vi "RecordWave_and_WAVFile.vi"() -> ()   [LabVIEW 2016]
uses:
  WaveIO.llb/SoundHandle.ctl
panel:
  in  "Write CSV":bool
  out "bufferTime [µs]":dbl format="%#_6f"
  out "Time[sec]":dbl
  out "About":string
  in  "Stop File":bool
  in  "time to record":u32=1000 min=10 max=60000 step=10
  out "bufNo":i32=337
  out "Sound Handle IN":T1={"DeviceID"=0, "Samples/buf"=2205, "Sampl rate"=44100, "Bits/sample"=16, "Channels"=2, "Opened"=TRUE}
  in  "Record File":bool
  in  "Name of WAV File":path=path "soundcard_data.wav"
  in  "card #":u32
  out "Device Names":string[](array[string])
  out "Number of Input Devices":i32=3
  out "error out":errorcluster
  out "Rec Error":errorcluster
  in  "Format":cluster{"Rate":i32, "Bits":i32, "Channels":i32}={"Rate"=44100, "Bits"=16, "Channels"=2}
  in  "Buffer":T2={"# buffers"=10, "Buffer size"=50, "unit (ms)"=enum."time (ms)"}
  out "Waveform Graph":i32[][](graph)
  in  "Stop":bool=TRUE
  # "msec"
  # "ONLY for Information\nHas no effect in the code !"
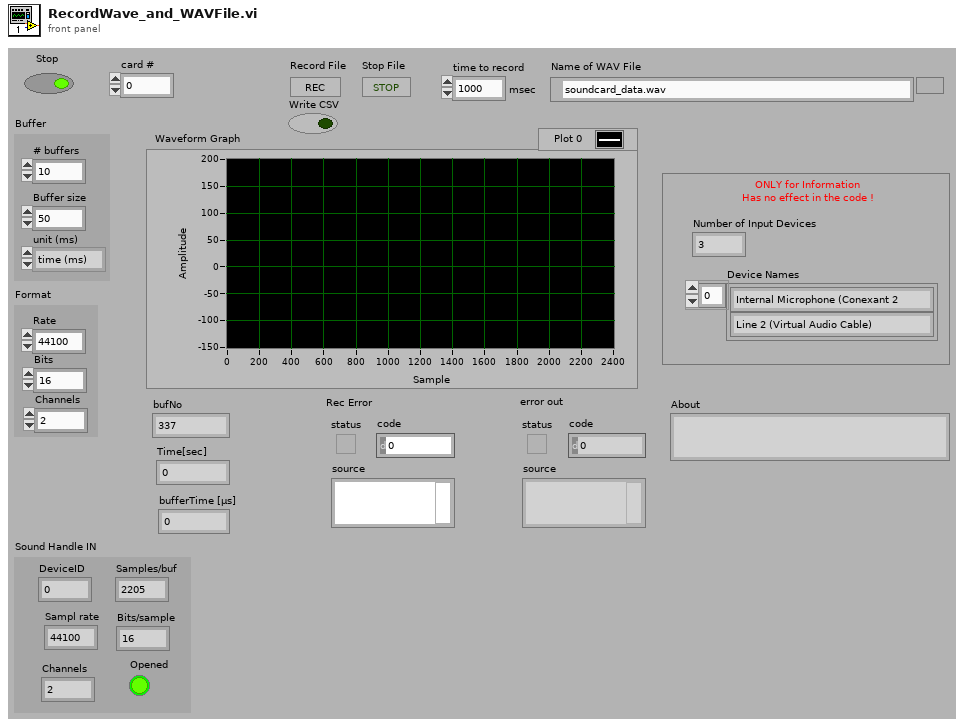
[diagram p1: front panel]
types:
  T1 = typedef "SoundHandle.ctl" = cluster{"DeviceID":u16, "Samples/buf":u32, "Sampl rate":u32, "Bits/sample":u16, "Channels":u8, "Opened":bool}
  T2 = cluster{"# buffers":i32, "Buffer size":i32, "unit (ms)":enum16{"time (ms)", "Samples"}}
  T3 = cluster{"active":bool, "WriteBuffer":bool, "Opened":bool, "Closing":bool}
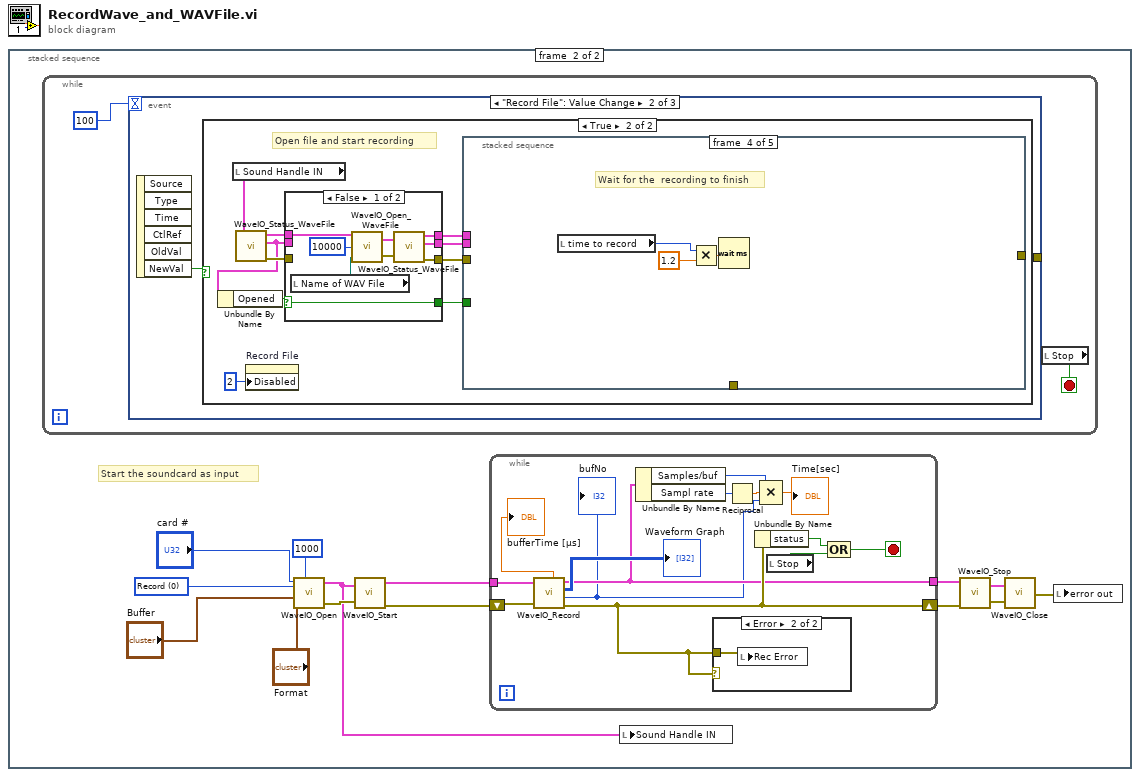
[diagram p0: block diagram]
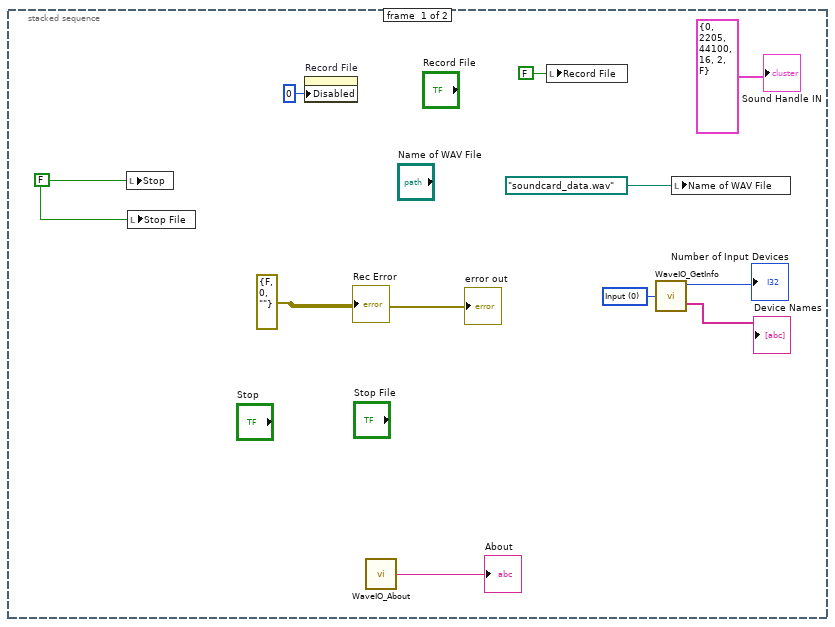
[diagram p2: hidden frame]
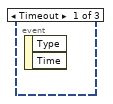
[diagram p4: hidden frame]
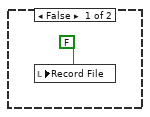
[diagram p5: hidden frame]
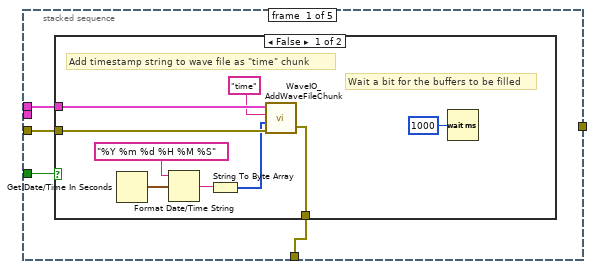
[diagram p7: hidden frame]
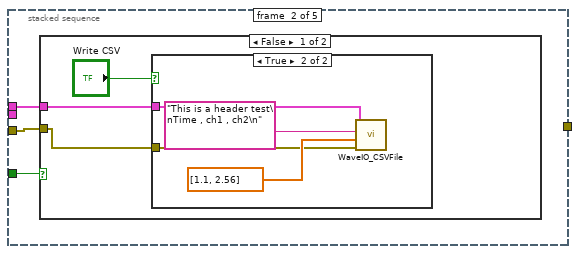
[diagram p9: hidden frame]
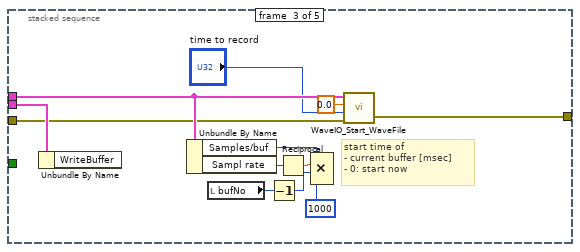
[diagram p12: hidden frame]
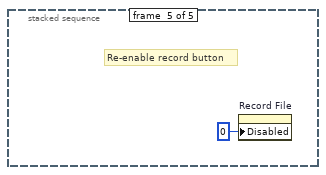
[diagram p13: hidden frame]
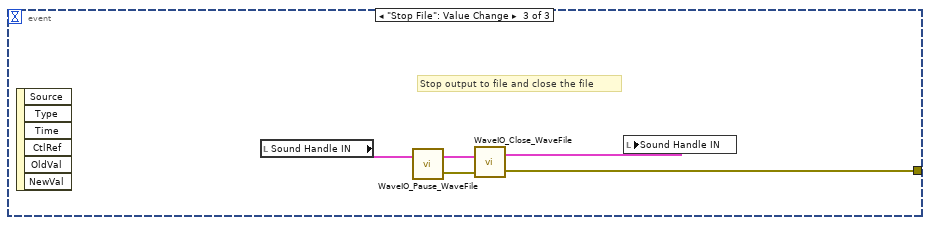
[diagram p14: hidden frame]
diagram:
  n1 = stacked-sequence {
    frame #0 {
      w5 = u16 0 items=["Input", "Output"] ("Direction (Input)")
      w10 = errorcluster {"status"=FALSE, "code"=0, "source"=""} ("error in (no error)")
      w4 = FALSE ("Stop")
      n2 = local write "Stop"(w4) -> ()
      n3 = local write "Stop File"(w4) -> ()
      n4 = property on="Record File" class="Bool (strict)"("Disabled"=u8 0) -> ()  [unwired: 2 in, 2 out]
      n5 = call "WaveIO_About.vi"() -> ("About"=→"About":string)  [unwired: 1 in]
      n6 = local write "Record File"(FALSE ("Record File")) -> ()
      n7 = call "WaveIO_GetInfo.vi"("Direction (Input)"=w5) -> ("numdev"=→"Number of Input Devices":i32, "Dev Names"=→"Device Names":string[])  [unwired: 2 out]
      n8 = local write "Name of WAV File"(path "soundcard_data.wav" ("Name of WAV File")) -> ()
      "Rec Error" <- w10
      "error out" <- w10
      "Sound Handle IN" <- T1 {"DeviceID"=0, "Samples/buf"=2205, "Sampl rate"=44100, "Bits/sample"=16, "Channels"=2, "Opened"=FALSE} ("Sound Handle IN")
    }
    frame #1 {
      w17 = u16 0 items=["Record", "Play"] ("Direction (Record)")
      # "Start the soundcard as input"
      n9 = while {
        stop <- w40 stop-if-true
        n10 = event shown="[1] \"Record File\": Value Change" {
          selector: _ -> [_ _ _]
          dyn-events: _ -> [_ _ _]
          timeout: 100 -> [_ _ _]
          tunnel: [_ _ w106] -> _
          event Timeout {
            n11 = event-data() -> ()  [unwired: 1 in, 2 out]
          }
          event "Record File": Value Change {
            n12 = event-data() -> ("NewVal"=w42:bool)  [unwired: 1 in, 5 out]
            n13 = case shown="True" w42 {
              frame False {
                n14 = local write "Record File"(FALSE ("Record File")) -> ()
              }
              frame True {
                # "Open file and start recording"
                n15 = local read "Sound Handle IN"() -> (w50:T1)
                n16 = call "WaveIO_Status_WaveFile.vi"("Handle"=w50) -> ("Handle Out"=w49:T1, "Status"=w47:T3, "error out"=w48:errorcluster)  [unwired: 1 in, 3 out]
                n17 = Unbundle By Name(w47) -> ("Opened"=w46:bool)
                n18 = property on="Record File" class="Bool (strict)"("Disabled"=u8 2) -> ()  [unwired: 2 in, 2 out]
                n19 = case shown="False" w46 {
                  selector: w46 -> [w54 _]
                  tunnel: [w60 w64] -> w53
                  tunnel: [w59 w63] -> w44
                  tunnel: [w58 w65] -> w52
                  tunnel: w49 -> [w55 w64]
                  tunnel: w47 -> [_ w65]
                  tunnel: w48 -> [_ w63]
                  tunnel: [w54 _] -> w45
                  frame False {
                    n20 = local read "Name of WAV File"() -> (w56:path)
                    n21 = call "WaveIO_Open_WaveFile.vi"("Wave File name"=w56, "Buffer length (ms)"=10000, "Sound Handle IN"=w55) -> ("error out"=w61:errorcluster, "Sound Handle Out"=w62:T1)
                    n22 = call "WaveIO_Status_WaveFile.vi"("Handle"=w62, "error in (no error)"=w61) -> ("Handle Out"=w60:T1, "Status"=w58:T3, "error out"=w59:errorcluster)  [unwired: 3 out]
                  }
                  frame True {
                  }
                }
                n23 = stacked-sequence {
                  tunnel: w53 -> [w69 w81 w100 _ _]
                  tunnel: w52 -> [_ _ w99 _ _]
                  tunnel: [w68 _ _ _ _] -> _
                  tunnel: w45 -> [w67 w80 _ _ _]
                  tunnel: [_ _ w91 _ _] -> _
                  tunnel: w44 -> [w66 w79 w89 _ _]
                  frame #0 {
                    n24 = case shown="False" w67 {
                      tunnel: w69 -> [w78 _]
                      tunnel: w66 -> [w77 _]
                      tunnel: [w71 _] -> w68
                      frame False {
                        # "Wait a bit for the buffers to be filled"
                        # "Add timestamp string to wave file as \"time\" chunk"
                        n25 = Get Date/Time In Seconds() -> (seconds since 1Jan1904=w76:timestamp)
                        n26 = Format Date/Time String(time format string (%c)="%Y %m %d %H %M %S", seconds (now)=w76) -> (date/time string=w73:string)  [unwired: 1 in]
                        n27 = String To Byte Array(string=w73) -> (unsigned byte array=w72:u8[])
                        n28 = call "WaveIO_AddWaveFileChunk.vi"("error in (no error)"=w77, "Data (<256 Bytes)"=w72, "Wave Chunk Name (4 chars)"="time", "Handle"=w78) -> ("error out"=w71:errorcluster)  [unwired: 1 out]
                        n29 = Wait (ms)(milliseconds to wait=u32 1000) -> ()  [unwired: 1 out]
                      }
                      frame True {
                      }
                    }
                  }
                  frame #1 {
                    n30 = case shown="False" w80 {
                      tunnel: w81 -> [w83 _]
                      tunnel: w79 -> [w82 _]
                      frame False {
                        n31 = case shown="True" "Write CSV" {
                          tunnel: w83 -> [_ w86]
                          tunnel: w82 -> [_ w85]
                          frame False {
                          }
                          frame True {
                            n32 = call "WaveIO_CSVFile.vi"("Sound Handle IN"=w86, "Header String"="This is a header test\nTime , ch1 , ch2\n" ("strHeader"), "Channel Scale Factors"=dbl[] [1.1, 2.56] ("calib"), "error in (no error)"=w85) -> ()  [unwired: 1 in, 2 out]
                          }
                        }
                      }
                      frame True {
                      }
                    }
                  }
                  frame #2 {
                    # "start time of \n- current buffer [msec]\n- 0: start now"
                    n33 = Unbundle By Name(w99) -> ()  [unwired: 1 out]
                    n34 = Unbundle By Name(w100) -> ("Samples/buf"=w98:u32, "Sampl rate"=w96:u32)
                    n35 = local read "bufNo"() -> (w97:i32)
                    n36 = Decrement(x=w97) -> (x-1=w92:i32)
                    n37 = Reciprocal(x=w96) -> (1/x=w94:dbl)
                    n38 = Compound Arithmetic op=MULTIPLY(w98, w94, w92, 1000 ("value")) -> ()  [unwired: 1 out]
                    n39 = call "WaveIO_Start_WaveFile.vi"("error in (no error)"=w89, "delta_t"="time to record", "Time"=0.0, "Handle"=w100) -> ("error out"=w91:errorcluster)  [unwired: 1 out]
                  }
                  frame #3 {
                    # "Wait for the  recording to finish"
                    n40 = local read "time to record"() -> (w103:u32)
                    n41 = Multiply(x=w103, y=1.2) -> (x*y=w102:dbl)
                    n42 = Wait (ms)(milliseconds to wait=w102) -> ()  [unwired: 1 out]
                  }
                  frame #4 {
                    # "Re-enable record button"
                    n43 = property on="Record File" class="Bool (strict)"("Disabled"=u8 0) -> ()  [unwired: 2 in, 2 out]
                  }
                }
              }
            }
          }
          event "Stop File": Value Change {
            # "Stop output to file and close the file"
            n44 = event-data() -> ()  [unwired: 1 in, 6 out]
            n45 = local read "Sound Handle IN"() -> (w109:T1)
            n46 = call "WaveIO_Pause_WaveFile.vi"("Handle"=w109) -> ("error out"=w107:errorcluster, "Handle Out"=w108:T1)  [unwired: 1 in]
            n47 = call "WaveIO_Close_WaveFile.vi"("error in (no error)"=w107, "Handle"=w108) -> ("error out"=w106:errorcluster, "Handle Out"=w105:T1)
            n48 = local write "Sound Handle IN"(w105) -> ()
          }
        }
        n49 = local read "Stop"() -> (w40:bool)
      }
      n50 = call "WaveIO_Open.vi"("idev"="card #", "Watchdog timeout (msec) (default=OFF)"=1000, "device type (Record)"=w17, "Buffer Config"="Buffer", "Format (44kHz, 16Bit, stereo)"="Format") -> ("Sound Handle Out"=w11:T1, "error out"=w21:errorcluster)  [unwired: 2 in]
      n51 = call "WaveIO_Start.vi"("error in (no error)"=w21, "Handle"=w11) -> ("error out"=w18:errorcluster, "Handle Out"=w19:T1)
      n52 = while {
        shift-right: [w33] -> w16
        shift-left: w18 -> [w36]
        tunnel: w19 -> [w37]
        tunnel: [w28] -> w23
        stop <- w32 stop-if-true
        n53 = call "WaveIO_Record.vi"("Handle"=w37, "error in (no error)"=w36) -> ("Handle Out"=w28:T1, "Data"=→"Waveform Graph":i32[][], "bufNo"=w27:i32, "error out"=w33:errorcluster, "bufferTime [µs]"=→"bufferTime [µs]":dbl)  [unwired: 1 in]
        "bufNo" <- w27
        n54 = Unbundle By Name(w28) -> ("Samples/buf"=w31:u32, "Sampl rate"=w30:u32)
        n55 = case shown="Error" w33 {
          tunnel: w33 -> [_ w39]
          frame No Error {
          }
          frame Error {
            n56 = local write "Rec Error"(w39) -> ()
          }
        }
        n57 = Reciprocal(x=w30) -> (1/x=w29:dbl)
        n58 = Unbundle By Name(w33) -> ("status"=w38:bool)
        n59 = Compound Arithmetic op=MULTIPLY(w31, w29, w27) -> (→"Time[sec]":dbl)
        n60 = local read "Stop"() -> (w35:bool)
        n61 = Compound Arithmetic op=OR(w38, w35) -> (w32:bool)
      }
      n62 = local write "Sound Handle IN"(w11) -> ()
      n63 = call "WaveIO_Stop.vi"("error in (no error)"=w16, "Handle"=w23) -> ("error out"=w20:errorcluster, "Handle Out"=w24:T1)
      n64 = call "WaveIO_Close.vi"("error in (no error)"=w20, "Handle"=w24) -> ("error out"=w12:errorcluster)  [unwired: 1 out]
      n65 = local write "error out"(w12) -> ()
    }
  }
